vi "Autonomous Independent.vi"   [LabVIEW 2019]
doc: "This VI is called when autonomous begins, and will automatically be terminated when autonomous ends. You can carry out timed or sensor driven robot movement independently without needing to return to the caller."
uses:
  <vilib>/Rock Robotics/WPI/Utilities/WPI_GetSetVariantRefNum.vi
  <vilib>/Rock Robotics/Network Tables/NT Read String.vi
  <vilib>/Rock Robotics/Network Tables/NT Write Numeric Array.vi
  Robot Global Data.vi
panel:
  # "Be sure to right-click and choose Data Operations>>Make Current Value default if you want to save the array values with the VI"
types:
  T1 = typedef "WPI_JoystickDevRef.ctl" = cluster{"Device":T2}
  T2 = typedef "WPI_JoystickDeviceEnum.ctl" = enum16{"USB 0", "USB 1", "USB 2", "USB 3", "USB 4", "USB 5"}
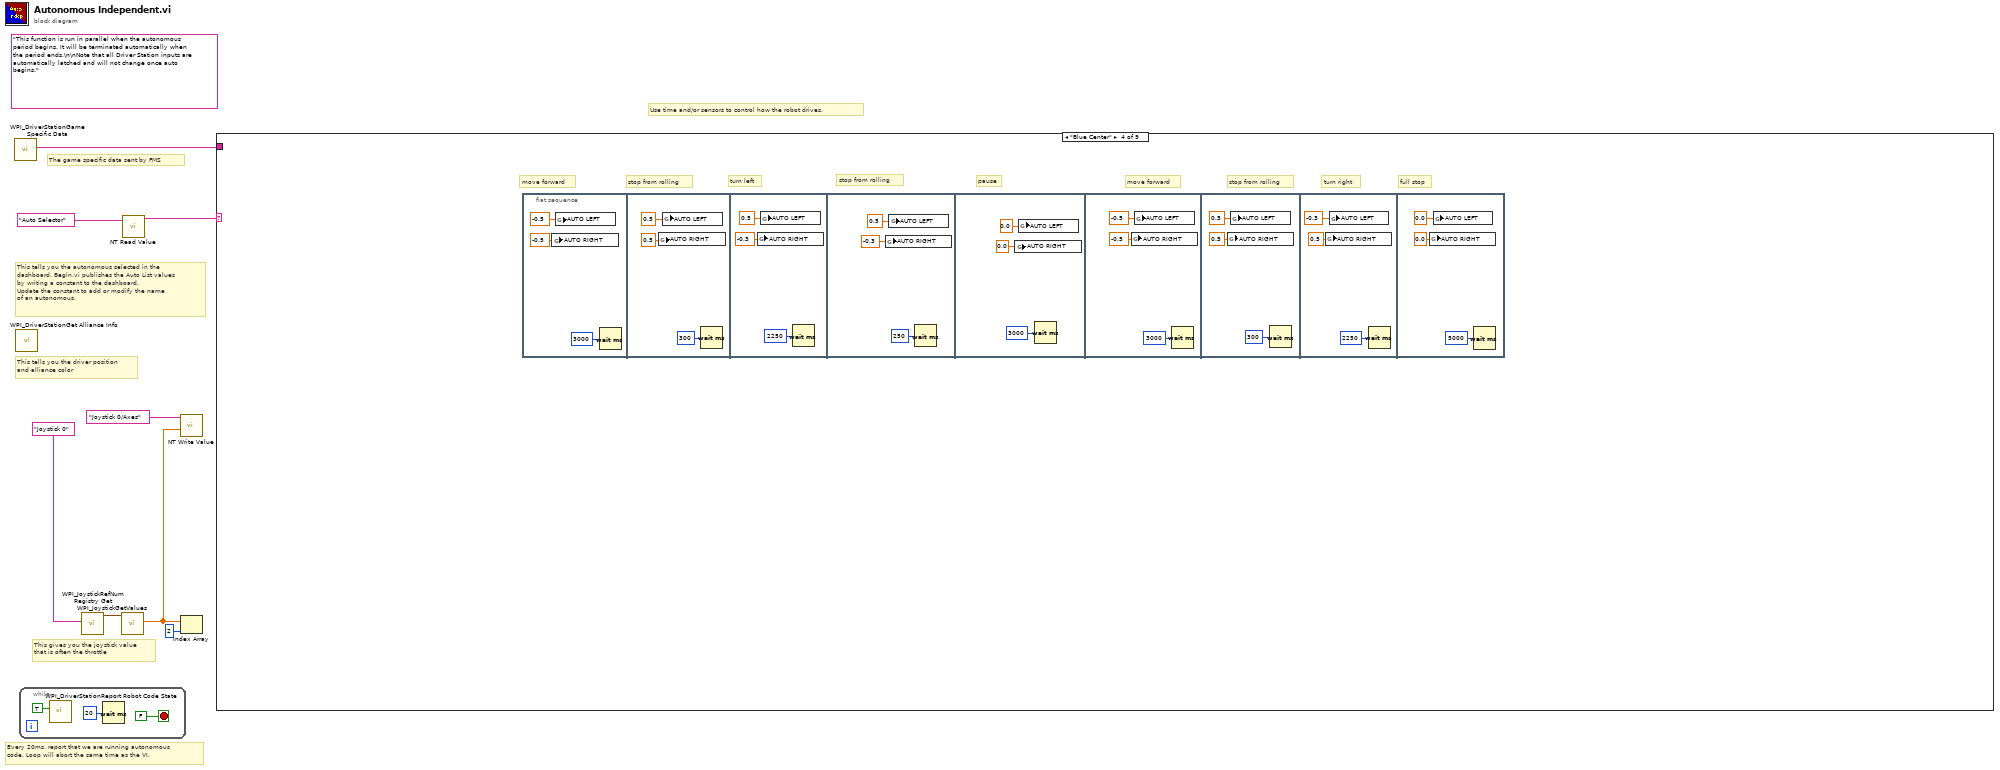
[diagram p0: block diagram]
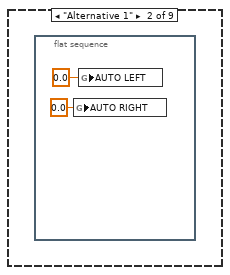
[diagram p3: hidden frame]
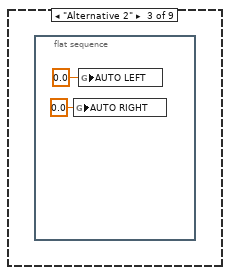
[diagram p4: hidden frame]
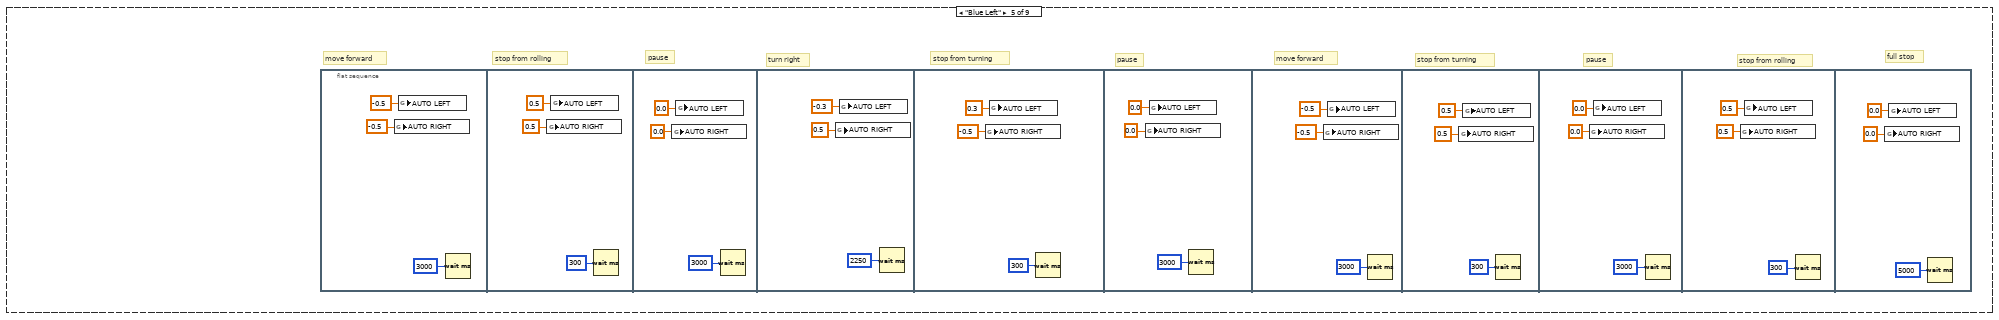
[diagram p5: hidden frame]
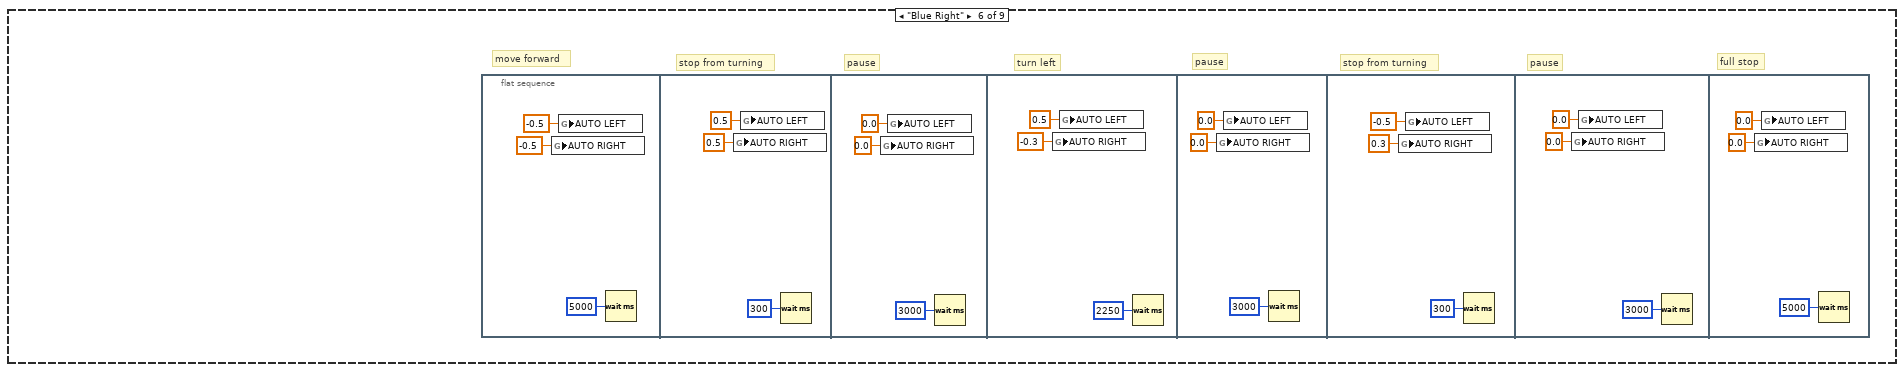
[diagram p6: hidden frame]
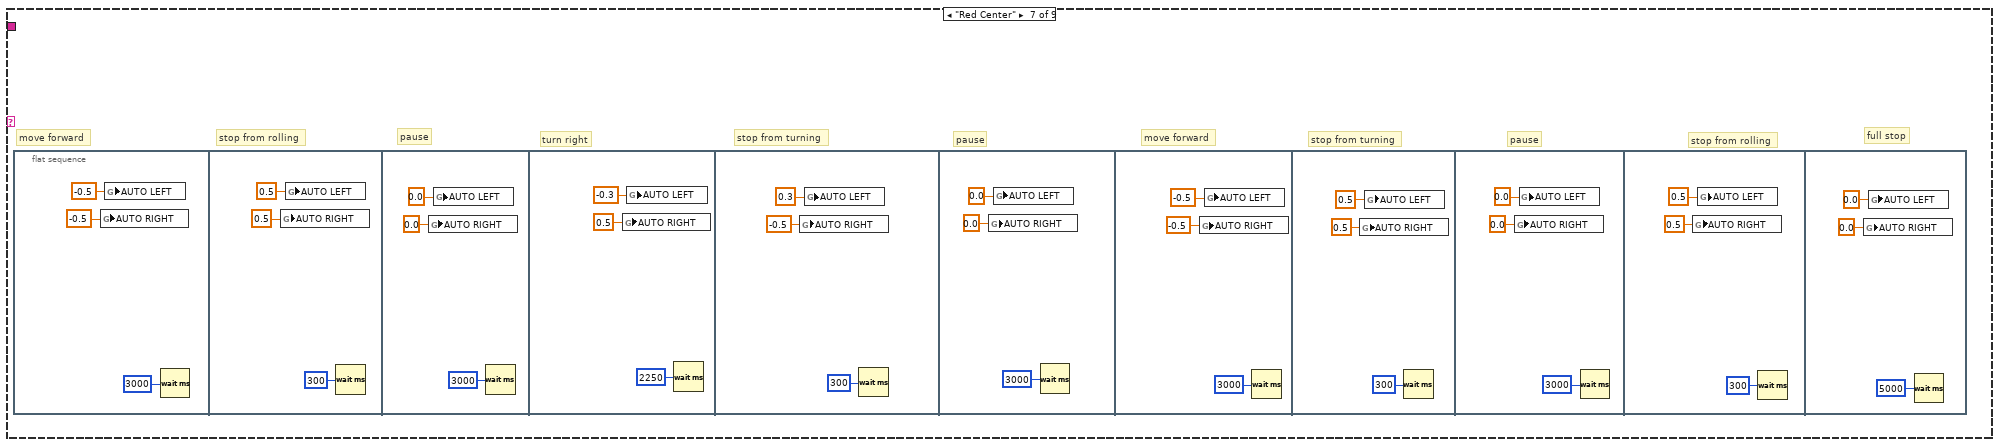
[diagram p7: hidden frame]
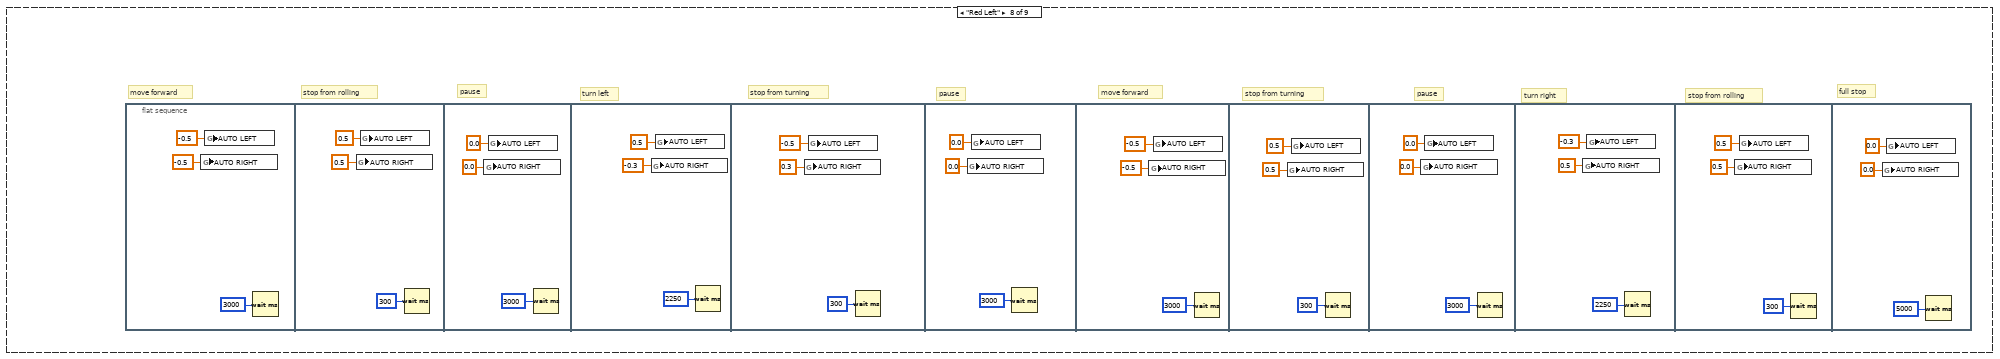
[diagram p8: hidden frame]
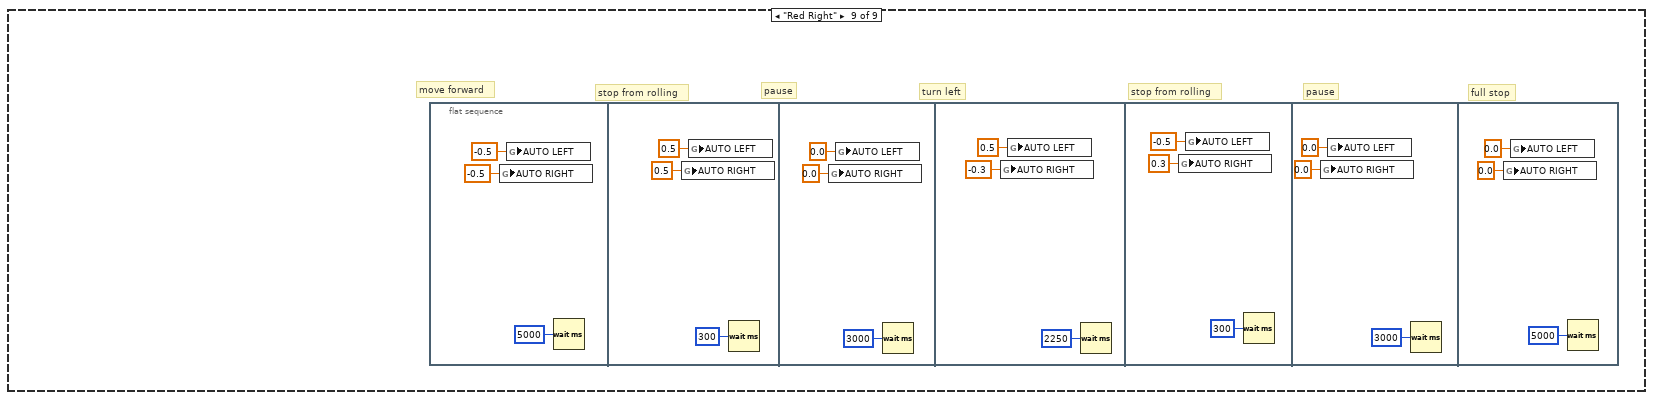
[diagram p9: hidden frame]
diagram:
  (unwired) "This function is run in parallel when the autonomous period begins. It will be terminated automatically when the period ends.\n\nNote that all Driver Station inputs are automatically latched and will not change once auto begins."
  # "The game specific data sent by FMS"
  # "This tells you the autonomous selected in the \ndashboard. Begin.vi publishes the Auto List values\nby writing a constant to the dashboard.\nUpdate the constant to add or modify the name\nof an autonomous."
  # "Every 20ms, report that we are running autonomous\ncode. Loop will abort the same time as the VI."
  # "This gives you the joystick value\nthat is often the throttle"
  # "Use time and/or sensors to control how the robot drives."
  # "This tells you the driver position\nand alliance color"
  n1 = call <vilib>:"WPI_DriverStationGame Specific Data.vi"() -> ("Game Specific Data"=w1:string)  [unwired: 11 in]
  n2 = call <vilib>:"WPI_DriverStationGet Alliance Info.vi"() -> ()  [unwired: 12 out]
  n3 = while {
    stop <- FALSE stop-if-true
    n4 = call <vilib>:"WPI_DriverStationReport Robot Code State.vi"("Autonomous"=TRUE) -> ()  [unwired: 10 in, 1 out]
    n5 = Wait (ms)(milliseconds to wait=u32 20) -> ()  [unwired: 1 out]
  }
  n6 = call <vilib>:"WPI_JoystickRefNum Registry Get.vi"("refnum name"="Joystick 0") -> ("JoystickDevRef"=w7:T1)  [unwired: 1 in, 9 out]
  n7 = call <vilib>:"WPI_JoystickGetValues.vi"("JoystickDevRef"=w7) -> ("Axes"=w3:dbl[])  [unwired: 6 in, 4 out]
  n8 = call-poly <vilib>:"NT Read Value.vi"("Name"="Auto Selector") -> ("String"=w4:string)  [unwired: 9 in, 1 out]
  n9 = call-poly <vilib>:"NT Write Value.vi"("Numeric Array"=w3, "Name"="Joystick 0/Axes") -> ()  [unwired: 9 in, 1 out]
  n10 = Index Array(array=w3, index=2) -> ()  [unwired: 1 out]
  n11 = case shown="\"Blue Center\"" w4 {
    tunnel: w1 -> [_ _ _ _ _ _ _ _ _]
    frame Default {
      # "You can put your main auto here, or you can right-click on the case and make any\nother frame be the default case."
      # "This is the frame that will execute if no selection is made, or if it is not recognized"
    }
    frame "Alternative 1" {
      n12 = flat-sequence {
        frame #0 {
          n13 = global write "Robot Global Data.vi" "AUTO RIGHT"(0.0 ("AUTO RIGHT")) -> ()
          n14 = global write "Robot Global Data.vi" "AUTO LEFT"(0.0 ("AUTO LEFT")) -> ()
        }
      }
    }
    frame "Alternative 2" {
      n15 = flat-sequence {
        frame #0 {
          n16 = global write "Robot Global Data.vi" "AUTO RIGHT"(0.0 ("AUTO RIGHT")) -> ()
          n17 = global write "Robot Global Data.vi" "AUTO LEFT"(0.0 ("AUTO LEFT")) -> ()
        }
      }
    }
    frame "Blue Center" {
      # "pause"
      # "stop from rolling"
      # "full stop"
      # "stop from rolling"
      # "turn right"
      # "move forward"
      # "turn left"
      # "stop from rolling"
      # "move forward"
      n18 = flat-sequence {
        frame #0 {
          n19 = global write "Robot Global Data.vi" "AUTO RIGHT"(-0.5 ("AUTO LEFT")) -> ()
          n20 = global write "Robot Global Data.vi" "AUTO LEFT"(-0.5 ("AUTO LEFT")) -> ()
          n21 = Wait (ms)(milliseconds to wait=u32 3000) -> ()  [unwired: 1 out]
        }
        frame #1 {
          n22 = global write "Robot Global Data.vi" "AUTO RIGHT"(0.5 ("AUTO LEFT")) -> ()
          n23 = global write "Robot Global Data.vi" "AUTO LEFT"(0.5 ("AUTO LEFT")) -> ()
          n24 = Wait (ms)(milliseconds to wait=u32 300) -> ()  [unwired: 1 out]
        }
        frame #2 {
          n25 = global write "Robot Global Data.vi" "AUTO RIGHT"(-0.3 ("AUTO LEFT")) -> ()
          n26 = global write "Robot Global Data.vi" "AUTO LEFT"(0.5 ("AUTO LEFT")) -> ()
          n27 = Wait (ms)(milliseconds to wait=u32 2250) -> ()  [unwired: 1 out]
        }
        frame #3 {
          n28 = global write "Robot Global Data.vi" "AUTO RIGHT"(-0.3 ("AUTO RIGHT")) -> ()
          n29 = global write "Robot Global Data.vi" "AUTO LEFT"(0.5 ("AUTO LEFT")) -> ()
          n30 = Wait (ms)(milliseconds to wait=u32 250) -> ()  [unwired: 1 out]
        }
        frame #4 {
          n31 = global write "Robot Global Data.vi" "AUTO RIGHT"(0.0 ("AUTO RIGHT")) -> ()
          n32 = global write "Robot Global Data.vi" "AUTO LEFT"(0.0 ("AUTO LEFT")) -> ()
          n33 = Wait (ms)(milliseconds to wait=u32 3000) -> ()  [unwired: 1 out]
        }
        frame #5 {
          n34 = global write "Robot Global Data.vi" "AUTO RIGHT"(-0.5 ("AUTO LEFT")) -> ()
          n35 = global write "Robot Global Data.vi" "AUTO LEFT"(-0.5 ("AUTO LEFT")) -> ()
          n36 = Wait (ms)(milliseconds to wait=u32 3000) -> ()  [unwired: 1 out]
        }
        frame #6 {
          n37 = global write "Robot Global Data.vi" "AUTO RIGHT"(0.5 ("AUTO LEFT")) -> ()
          n38 = global write "Robot Global Data.vi" "AUTO LEFT"(0.5 ("AUTO LEFT")) -> ()
          n39 = Wait (ms)(milliseconds to wait=u32 300) -> ()  [unwired: 1 out]
        }
        frame #7 {
          n40 = global write "Robot Global Data.vi" "AUTO RIGHT"(0.5 ("AUTO LEFT")) -> ()
          n41 = global write "Robot Global Data.vi" "AUTO LEFT"(-0.3 ("AUTO LEFT")) -> ()
          n42 = Wait (ms)(milliseconds to wait=u32 2250) -> ()  [unwired: 1 out]
        }
        frame #8 {
          n43 = global write "Robot Global Data.vi" "AUTO RIGHT"(0.0 ("AUTO LEFT")) -> ()
          n44 = global write "Robot Global Data.vi" "AUTO LEFT"(0.0 ("AUTO LEFT")) -> ()
          n45 = Wait (ms)(milliseconds to wait=u32 5000) -> ()  [unwired: 1 out]
        }
      }
    }
    frame "Blue Left" {
      # "stop from turning"
      # "pause"
      # "pause"
      # "pause"
      # "full stop"
      # "stop from rolling"
      # "move forward"
      # "stop from turning"
      # "turn right"
      # "stop from rolling"
      # "move forward"
      n46 = flat-sequence {
        frame #0 {
          n47 = global write "Robot Global Data.vi" "AUTO RIGHT"(-0.5 ("AUTO RIGHT")) -> ()
          n48 = global write "Robot Global Data.vi" "AUTO LEFT"(-0.5 ("AUTO LEFT")) -> ()
          n49 = Wait (ms)(milliseconds to wait=u32 3000) -> ()  [unwired: 1 out]
        }
        frame #1 {
          n50 = global write "Robot Global Data.vi" "AUTO RIGHT"(0.5 ("AUTO RIGHT")) -> ()
          n51 = global write "Robot Global Data.vi" "AUTO LEFT"(0.5 ("AUTO LEFT")) -> ()
          n52 = Wait (ms)(milliseconds to wait=u32 300) -> ()  [unwired: 1 out]
        }
        frame #2 {
          n53 = global write "Robot Global Data.vi" "AUTO RIGHT"(0.0 ("AUTO RIGHT")) -> ()
          n54 = global write "Robot Global Data.vi" "AUTO LEFT"(0.0 ("AUTO LEFT")) -> ()
          n55 = Wait (ms)(milliseconds to wait=u32 3000) -> ()  [unwired: 1 out]
        }
        frame #3 {
          n56 = global write "Robot Global Data.vi" "AUTO RIGHT"(0.5 ("AUTO RIGHT")) -> ()
          n57 = global write "Robot Global Data.vi" "AUTO LEFT"(-0.3 ("AUTO LEFT")) -> ()
          n58 = Wait (ms)(milliseconds to wait=u32 2250) -> ()  [unwired: 1 out]
        }
        frame #4 {
          n59 = global write "Robot Global Data.vi" "AUTO RIGHT"(-0.5 ("AUTO RIGHT")) -> ()
          n60 = global write "Robot Global Data.vi" "AUTO LEFT"(0.3 ("AUTO LEFT")) -> ()
          n61 = Wait (ms)(milliseconds to wait=u32 300) -> ()  [unwired: 1 out]
        }
        frame #5 {
          n62 = global write "Robot Global Data.vi" "AUTO RIGHT"(0.0 ("AUTO RIGHT")) -> ()
          n63 = global write "Robot Global Data.vi" "AUTO LEFT"(0.0 ("AUTO LEFT")) -> ()
          n64 = Wait (ms)(milliseconds to wait=u32 3000) -> ()  [unwired: 1 out]
        }
        frame #6 {
          n65 = global write "Robot Global Data.vi" "AUTO RIGHT"(-0.5 ("AUTO RIGHT")) -> ()
          n66 = global write "Robot Global Data.vi" "AUTO LEFT"(-0.5 ("AUTO LEFT")) -> ()
          n67 = Wait (ms)(milliseconds to wait=u32 3000) -> ()  [unwired: 1 out]
        }
        frame #7 {
          n68 = global write "Robot Global Data.vi" "AUTO RIGHT"(0.5 ("AUTO RIGHT")) -> ()
          n69 = global write "Robot Global Data.vi" "AUTO LEFT"(0.5 ("AUTO LEFT")) -> ()
          n70 = Wait (ms)(milliseconds to wait=u32 300) -> ()  [unwired: 1 out]
        }
        frame #8 {
          n71 = global write "Robot Global Data.vi" "AUTO RIGHT"(0.0 ("AUTO RIGHT")) -> ()
          n72 = global write "Robot Global Data.vi" "AUTO LEFT"(0.0 ("AUTO LEFT")) -> ()
          n73 = Wait (ms)(milliseconds to wait=u32 3000) -> ()  [unwired: 1 out]
        }
        frame #9 {
          n74 = global write "Robot Global Data.vi" "AUTO RIGHT"(0.5 ("AUTO RIGHT")) -> ()
          n75 = global write "Robot Global Data.vi" "AUTO LEFT"(0.5 ("AUTO LEFT")) -> ()
          n76 = Wait (ms)(milliseconds to wait=u32 300) -> ()  [unwired: 1 out]
        }
        frame #10 {
          n77 = global write "Robot Global Data.vi" "AUTO RIGHT"(0.0 ("AUTO RIGHT")) -> ()
          n78 = global write "Robot Global Data.vi" "AUTO LEFT"(0.0 ("AUTO LEFT")) -> ()
          n79 = Wait (ms)(milliseconds to wait=u32 5000) -> ()  [unwired: 1 out]
        }
      }
    }
    frame "Blue Right" {
      # "full stop"
      # "pause"
      # "pause"
      # "pause"
      # "stop from turning"
      # "turn left"
      # "stop from turning"
      # "move forward"
      n80 = flat-sequence {
        frame #0 {
          n81 = global write "Robot Global Data.vi" "AUTO RIGHT"(-0.5 ("AUTO RIGHT")) -> ()
          n82 = global write "Robot Global Data.vi" "AUTO LEFT"(-0.5 ("AUTO LEFT")) -> ()
          n83 = Wait (ms)(milliseconds to wait=u32 5000) -> ()  [unwired: 1 out]
        }
        frame #1 {
          n84 = global write "Robot Global Data.vi" "AUTO RIGHT"(0.5 ("AUTO RIGHT")) -> ()
          n85 = global write "Robot Global Data.vi" "AUTO LEFT"(0.5 ("AUTO LEFT")) -> ()
          n86 = Wait (ms)(milliseconds to wait=u32 300) -> ()  [unwired: 1 out]
        }
        frame #2 {
          n87 = global write "Robot Global Data.vi" "AUTO RIGHT"(0.0 ("AUTO RIGHT")) -> ()
          n88 = global write "Robot Global Data.vi" "AUTO LEFT"(0.0 ("AUTO LEFT")) -> ()
          n89 = Wait (ms)(milliseconds to wait=u32 3000) -> ()  [unwired: 1 out]
        }
        frame #3 {
          n90 = global write "Robot Global Data.vi" "AUTO RIGHT"(-0.3 ("AUTO RIGHT")) -> ()
          n91 = global write "Robot Global Data.vi" "AUTO LEFT"(0.5 ("AUTO LEFT")) -> ()
          n92 = Wait (ms)(milliseconds to wait=u32 2250) -> ()  [unwired: 1 out]
        }
        frame #4 {
          n93 = global write "Robot Global Data.vi" "AUTO RIGHT"(0.0 ("AUTO RIGHT")) -> ()
          n94 = global write "Robot Global Data.vi" "AUTO LEFT"(0.0 ("AUTO LEFT")) -> ()
          n95 = Wait (ms)(milliseconds to wait=u32 3000) -> ()  [unwired: 1 out]
        }
        frame #5 {
          n96 = global write "Robot Global Data.vi" "AUTO RIGHT"(0.3 ("AUTO RIGHT")) -> ()
          n97 = global write "Robot Global Data.vi" "AUTO LEFT"(-0.5 ("AUTO LEFT")) -> ()
          n98 = Wait (ms)(milliseconds to wait=u32 300) -> ()  [unwired: 1 out]
        }
        frame #6 {
          n99 = global write "Robot Global Data.vi" "AUTO RIGHT"(0.0 ("AUTO RIGHT")) -> ()
          n100 = global write "Robot Global Data.vi" "AUTO LEFT"(0.0 ("AUTO LEFT")) -> ()
          n101 = Wait (ms)(milliseconds to wait=u32 3000) -> ()  [unwired: 1 out]
        }
        frame #7 {
          n102 = global write "Robot Global Data.vi" "AUTO RIGHT"(0.0 ("AUTO RIGHT")) -> ()
          n103 = global write "Robot Global Data.vi" "AUTO LEFT"(0.0 ("AUTO LEFT")) -> ()
          n104 = Wait (ms)(milliseconds to wait=u32 5000) -> ()  [unwired: 1 out]
        }
      }
    }
    frame "Red Center" {
      # "stop from turning"
      # "pause"
      # "pause"
      # "pause"
      # "full stop"
      # "stop from rolling"
      # "move forward"
      # "stop from turning"
      # "turn right"
      # "stop from rolling"
      # "move forward"
      n105 = flat-sequence {
        frame #0 {
          n106 = global write "Robot Global Data.vi" "AUTO RIGHT"(-0.5 ("AUTO RIGHT")) -> ()
          n107 = global write "Robot Global Data.vi" "AUTO LEFT"(-0.5 ("AUTO LEFT")) -> ()
          n108 = Wait (ms)(milliseconds to wait=u32 3000) -> ()  [unwired: 1 out]
        }
        frame #1 {
          n109 = global write "Robot Global Data.vi" "AUTO RIGHT"(0.5 ("AUTO RIGHT")) -> ()
          n110 = global write "Robot Global Data.vi" "AUTO LEFT"(0.5 ("AUTO LEFT")) -> ()
          n111 = Wait (ms)(milliseconds to wait=u32 300) -> ()  [unwired: 1 out]
        }
        frame #2 {
          n112 = global write "Robot Global Data.vi" "AUTO RIGHT"(0.0 ("AUTO RIGHT")) -> ()
          n113 = global write "Robot Global Data.vi" "AUTO LEFT"(0.0 ("AUTO LEFT")) -> ()
          n114 = Wait (ms)(milliseconds to wait=u32 3000) -> ()  [unwired: 1 out]
        }
        frame #3 {
          n115 = global write "Robot Global Data.vi" "AUTO RIGHT"(0.5 ("AUTO RIGHT")) -> ()
          n116 = global write "Robot Global Data.vi" "AUTO LEFT"(-0.3 ("AUTO LEFT")) -> ()
          n117 = Wait (ms)(milliseconds to wait=u32 2250) -> ()  [unwired: 1 out]
        }
        frame #4 {
          n118 = global write "Robot Global Data.vi" "AUTO RIGHT"(-0.5 ("AUTO RIGHT")) -> ()
          n119 = global write "Robot Global Data.vi" "AUTO LEFT"(0.3 ("AUTO LEFT")) -> ()
          n120 = Wait (ms)(milliseconds to wait=u32 300) -> ()  [unwired: 1 out]
        }
        frame #5 {
          n121 = global write "Robot Global Data.vi" "AUTO RIGHT"(0.0 ("AUTO RIGHT")) -> ()
          n122 = global write "Robot Global Data.vi" "AUTO LEFT"(0.0 ("AUTO LEFT")) -> ()
          n123 = Wait (ms)(milliseconds to wait=u32 3000) -> ()  [unwired: 1 out]
        }
        frame #6 {
          n124 = global write "Robot Global Data.vi" "AUTO RIGHT"(-0.5 ("AUTO RIGHT")) -> ()
          n125 = global write "Robot Global Data.vi" "AUTO LEFT"(-0.5 ("AUTO LEFT")) -> ()
          n126 = Wait (ms)(milliseconds to wait=u32 3000) -> ()  [unwired: 1 out]
        }
        frame #7 {
          n127 = global write "Robot Global Data.vi" "AUTO RIGHT"(0.5 ("AUTO RIGHT")) -> ()
          n128 = global write "Robot Global Data.vi" "AUTO LEFT"(0.5 ("AUTO LEFT")) -> ()
          n129 = Wait (ms)(milliseconds to wait=u32 300) -> ()  [unwired: 1 out]
        }
        frame #8 {
          n130 = global write "Robot Global Data.vi" "AUTO RIGHT"(0.0 ("AUTO RIGHT")) -> ()
          n131 = global write "Robot Global Data.vi" "AUTO LEFT"(0.0 ("AUTO LEFT")) -> ()
          n132 = Wait (ms)(milliseconds to wait=u32 3000) -> ()  [unwired: 1 out]
        }
        frame #9 {
          n133 = global write "Robot Global Data.vi" "AUTO RIGHT"(0.5 ("AUTO RIGHT")) -> ()
          n134 = global write "Robot Global Data.vi" "AUTO LEFT"(0.5 ("AUTO LEFT")) -> ()
          n135 = Wait (ms)(milliseconds to wait=u32 300) -> ()  [unwired: 1 out]
        }
        frame #10 {
          n136 = global write "Robot Global Data.vi" "AUTO RIGHT"(0.0 ("AUTO RIGHT")) -> ()
          n137 = global write "Robot Global Data.vi" "AUTO LEFT"(0.0 ("AUTO LEFT")) -> ()
          n138 = Wait (ms)(milliseconds to wait=u32 5000) -> ()  [unwired: 1 out]
        }
      }
    }
    frame "Red Left" {
      # "turn right"
      # "stop from turning"
      # "pause"
      # "pause"
      # "pause"
      # "full stop"
      # "stop from rolling"
      # "move forward"
      # "stop from turning"
      # "turn left"
      # "stop from rolling"
      # "move forward"
      n139 = flat-sequence {
        frame #0 {
          n140 = global write "Robot Global Data.vi" "AUTO RIGHT"(-0.5 ("AUTO RIGHT")) -> ()
          n141 = global write "Robot Global Data.vi" "AUTO LEFT"(-0.5 ("AUTO LEFT")) -> ()
          n142 = Wait (ms)(milliseconds to wait=u32 3000) -> ()  [unwired: 1 out]
        }
        frame #1 {
          n143 = global write "Robot Global Data.vi" "AUTO RIGHT"(0.5 ("AUTO RIGHT")) -> ()
          n144 = global write "Robot Global Data.vi" "AUTO LEFT"(0.5 ("AUTO LEFT")) -> ()
          n145 = Wait (ms)(milliseconds to wait=u32 300) -> ()  [unwired: 1 out]
        }
        frame #2 {
          n146 = global write "Robot Global Data.vi" "AUTO RIGHT"(0.0 ("AUTO RIGHT")) -> ()
          n147 = global write "Robot Global Data.vi" "AUTO LEFT"(0.0 ("AUTO LEFT")) -> ()
          n148 = Wait (ms)(milliseconds to wait=u32 3000) -> ()  [unwired: 1 out]
        }
        frame #3 {
          n149 = global write "Robot Global Data.vi" "AUTO RIGHT"(-0.3 ("AUTO RIGHT")) -> ()
          n150 = global write "Robot Global Data.vi" "AUTO LEFT"(0.5 ("AUTO LEFT")) -> ()
          n151 = Wait (ms)(milliseconds to wait=u32 2250) -> ()  [unwired: 1 out]
        }
        frame #4 {
          n152 = global write "Robot Global Data.vi" "AUTO RIGHT"(0.3 ("AUTO RIGHT")) -> ()
          n153 = global write "Robot Global Data.vi" "AUTO LEFT"(-0.5 ("AUTO LEFT")) -> ()
          n154 = Wait (ms)(milliseconds to wait=u32 300) -> ()  [unwired: 1 out]
        }
        frame #5 {
          n155 = global write "Robot Global Data.vi" "AUTO RIGHT"(0.0 ("AUTO RIGHT")) -> ()
          n156 = global write "Robot Global Data.vi" "AUTO LEFT"(0.0 ("AUTO LEFT")) -> ()
          n157 = Wait (ms)(milliseconds to wait=u32 3000) -> ()  [unwired: 1 out]
        }
        frame #6 {
          n158 = global write "Robot Global Data.vi" "AUTO RIGHT"(-0.5 ("AUTO RIGHT")) -> ()
          n159 = global write "Robot Global Data.vi" "AUTO LEFT"(-0.5 ("AUTO LEFT")) -> ()
          n160 = Wait (ms)(milliseconds to wait=u32 3000) -> ()  [unwired: 1 out]
        }
        frame #7 {
          n161 = global write "Robot Global Data.vi" "AUTO RIGHT"(0.5 ("AUTO RIGHT")) -> ()
          n162 = global write "Robot Global Data.vi" "AUTO LEFT"(0.5 ("AUTO LEFT")) -> ()
          n163 = Wait (ms)(milliseconds to wait=u32 300) -> ()  [unwired: 1 out]
        }
        frame #8 {
          n164 = global write "Robot Global Data.vi" "AUTO RIGHT"(0.0 ("AUTO RIGHT")) -> ()
          n165 = global write "Robot Global Data.vi" "AUTO LEFT"(0.0 ("AUTO LEFT")) -> ()
          n166 = Wait (ms)(milliseconds to wait=u32 3000) -> ()  [unwired: 1 out]
        }
        frame #9 {
          n167 = global write "Robot Global Data.vi" "AUTO RIGHT"(0.5 ("AUTO RIGHT")) -> ()
          n168 = global write "Robot Global Data.vi" "AUTO LEFT"(-0.3 ("AUTO LEFT")) -> ()
          n169 = Wait (ms)(milliseconds to wait=u32 2250) -> ()  [unwired: 1 out]
        }
        frame #10 {
          n170 = global write "Robot Global Data.vi" "AUTO RIGHT"(0.5 ("AUTO RIGHT")) -> ()
          n171 = global write "Robot Global Data.vi" "AUTO LEFT"(0.5 ("AUTO LEFT")) -> ()
          n172 = Wait (ms)(milliseconds to wait=u32 300) -> ()  [unwired: 1 out]
        }
        frame #11 {
          n173 = global write "Robot Global Data.vi" "AUTO RIGHT"(0.0 ("AUTO RIGHT")) -> ()
          n174 = global write "Robot Global Data.vi" "AUTO LEFT"(0.0 ("AUTO LEFT")) -> ()
          n175 = Wait (ms)(milliseconds to wait=u32 5000) -> ()  [unwired: 1 out]
        }
      }
    }
    frame "Red Right" {
      # "full stop"
      # "pause"
      # "stop from rolling"
      # "turn left"
      # "pause"
      # "stop from rolling"
      # "move forward"
      n176 = flat-sequence {
        frame #0 {
          n177 = global write "Robot Global Data.vi" "AUTO RIGHT"(-0.5 ("AUTO RIGHT")) -> ()
          n178 = global write "Robot Global Data.vi" "AUTO LEFT"(-0.5 ("AUTO LEFT")) -> ()
          n179 = Wait (ms)(milliseconds to wait=u32 5000) -> ()  [unwired: 1 out]
        }
        frame #1 {
          n180 = global write "Robot Global Data.vi" "AUTO RIGHT"(0.5 ("AUTO RIGHT")) -> ()
          n181 = global write "Robot Global Data.vi" "AUTO LEFT"(0.5 ("AUTO LEFT")) -> ()
          n182 = Wait (ms)(milliseconds to wait=u32 300) -> ()  [unwired: 1 out]
        }
        frame #2 {
          n183 = global write "Robot Global Data.vi" "AUTO RIGHT"(0.0 ("AUTO RIGHT")) -> ()
          n184 = global write "Robot Global Data.vi" "AUTO LEFT"(0.0 ("AUTO LEFT")) -> ()
          n185 = Wait (ms)(milliseconds to wait=u32 3000) -> ()  [unwired: 1 out]
        }
        frame #3 {
          n186 = global write "Robot Global Data.vi" "AUTO RIGHT"(-0.3 ("AUTO RIGHT")) -> ()
          n187 = global write "Robot Global Data.vi" "AUTO LEFT"(0.5 ("AUTO LEFT")) -> ()
          n188 = Wait (ms)(milliseconds to wait=u32 2250) -> ()  [unwired: 1 out]
        }
        frame #4 {
          n189 = global write "Robot Global Data.vi" "AUTO RIGHT"(0.3 ("AUTO RIGHT")) -> ()
          n190 = global write "Robot Global Data.vi" "AUTO LEFT"(-0.5 ("AUTO LEFT")) -> ()
          n191 = Wait (ms)(milliseconds to wait=u32 300) -> ()  [unwired: 1 out]
        }
        frame #5 {
          n192 = global write "Robot Global Data.vi" "AUTO RIGHT"(0.0 ("AUTO RIGHT")) -> ()
          n193 = global write "Robot Global Data.vi" "AUTO LEFT"(0.0 ("AUTO LEFT")) -> ()
          n194 = Wait (ms)(milliseconds to wait=u32 3000) -> ()  [unwired: 1 out]
        }
        frame #6 {
          n195 = global write "Robot Global Data.vi" "AUTO RIGHT"(0.0 ("AUTO RIGHT")) -> ()
          n196 = global write "Robot Global Data.vi" "AUTO LEFT"(0.0 ("AUTO LEFT")) -> ()
          n197 = Wait (ms)(milliseconds to wait=u32 5000) -> ()  [unwired: 1 out]
        }
      }
    }
  }
